vi "Check mtcdt check sd card write test.vi"(6 "VISA resource name":refnum<visa-resource-name>="COM5", 7 "Passed so far":bool, 8 "error in (no error)":errorcluster) -> (0 "error out":errorcluster, 1 "Card response":string, 2 "Source Response":string, 4 "VISA Refnum out":refnum<visa-resource-name>, 5 "Passed?":bool)   [LabVIEW 2024]
panel:
  out "Found sd card?":bool
  out "dest cksum":string
  out "src cksum":string
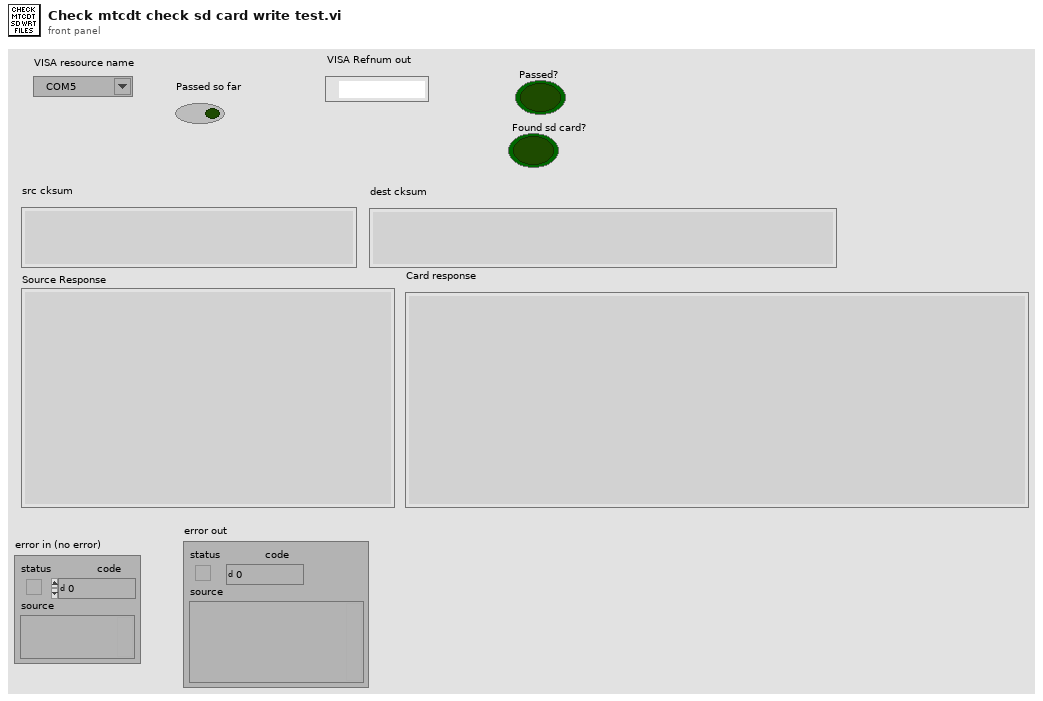
[diagram p1: front panel]
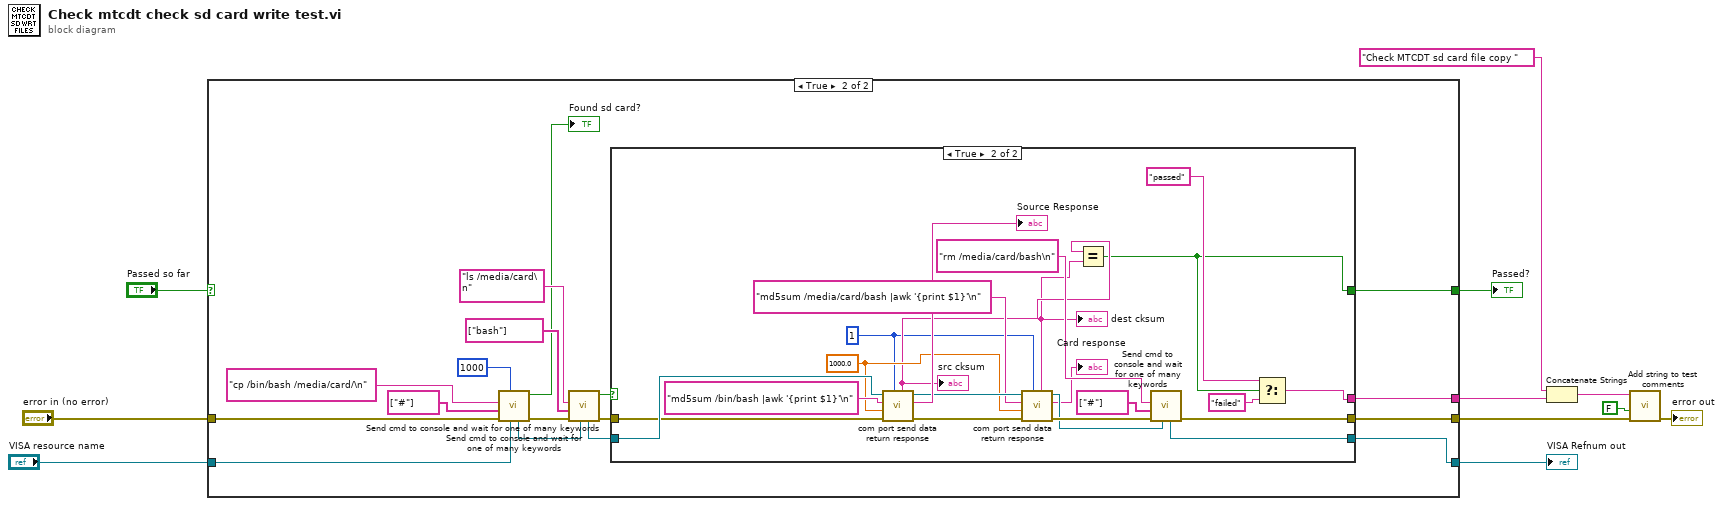
[diagram p0: block diagram]
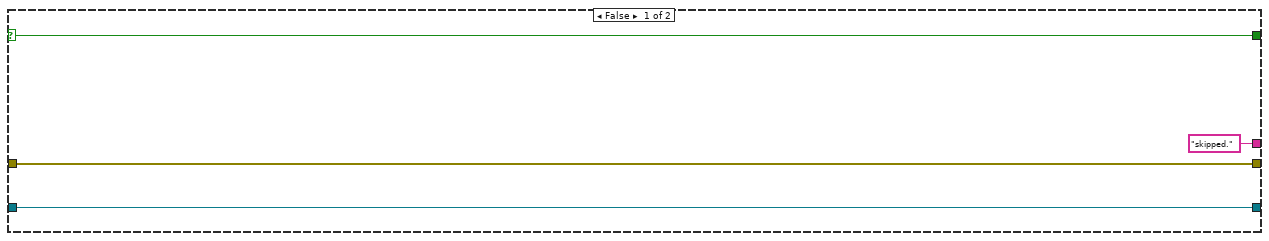
[diagram p2: hidden frame]
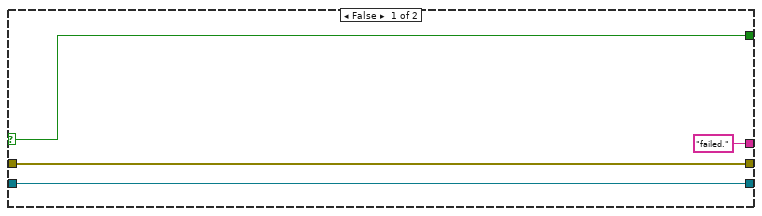
[diagram p3: hidden frame]
diagram:
  n1 = case shown="True" "Passed so far" {
    selector: "Passed so far" -> [w15 _]
    tunnel: "error in (no error)" -> [w14 w32]
    tunnel: [w14 w20] -> w2
    tunnel: "VISA resource name" -> [w13 w30]
    tunnel: [w15 w19] -> w6
    tunnel: [w13 w21] -> w3
    tunnel: ["skipped." w16] -> w1
    frame False {
    }
    frame True {
      n2 = call "Send cmd to console and wait for one of many keywords.vi"("VISA resource name"=w30, "Timeout (1000 mSecs)"=u32 1000 ("Timeout (mSecs)"), "error in (no error)"=w32, "Wait for keywords"=string[] ["#"], "write buffer"="cp /bin/bash /media/card/\n") -> ("error out"=w18:errorcluster, "Found key?"=→"Found sd card?":bool, "VISA Refnum out"=w27:refnum<visa-resource-name>)  [unwired: 2 in, 2 out]
      n3 = call "Send cmd to console and wait for one of many keywords.vi"("VISA resource name"=w27, "error in (no error)"=w18, "Wait for keywords"=string[] ["bash"], "write buffer"="ls /media/card\n") -> ("error out"=w23:errorcluster, "Found key?"=w24:bool, "VISA Refnum out"=w22:refnum<visa-resource-name>)  [unwired: 3 in, 2 out]
      n4 = case shown="True" w24 {
        selector: w24 -> [w34 _]
        tunnel: w23 -> [w36 w54]
        tunnel: w22 -> [w35 w55]
        tunnel: [w36 w57] -> w20
        tunnel: [w34 w38] -> w19
        tunnel: [w35 w56] -> w21
        tunnel: ["failed." w37] -> w16
        frame False {
        }
        frame True {
          w46 = u32 1 ("Return line number")
          w48 = 1000.0 ("Wait Msecs for response")
          n5 = call "com port send data return response.vi"("Return line number"=w46, "error in (no error)"=w54, "Wait Msecs for response"=w48, "Send data"="md5sum /bin/bash |awk '{print $1}'\n", "VISA resource name"=w55) -> ("error out"=w51:errorcluster, "response"=→"Source Response":string, "VISA resource name out"=w50:refnum<visa-resource-name>, "Response Line"=w47:string)  [unwired: 2 in, 1 out]
          "src cksum" <- w47
          n6 = call "com port send data return response.vi"("Return line number"=w46, "error in (no error)"=w51, "Wait Msecs for response"=w48, "Send data"="md5sum /media/card/bash |awk '{print $1}'\n", "VISA resource name"=w50) -> ("error out"=w44:errorcluster, "response"=→"Card response":string, "VISA resource name out"=w43:refnum<visa-resource-name>, "Response Line"=w45:string)  [unwired: 2 in, 1 out]
          "dest cksum" <- w45
          n7 = Equal?(x=w47, y=w45) -> (x = y?=w38:bool)
          n8 = call "Send cmd to console and wait for one of many keywords.vi"("VISA resource name"=w43, "error in (no error)"=w44, "Wait for keywords"=string[] ["#"], "write buffer"="rm /media/card/bash\n") -> ("error out"=w57:errorcluster, "VISA Refnum out"=w56:refnum<visa-resource-name>)  [unwired: 3 in, 3 out]
          n9 = Select(t="passed", s=w38, f="failed") -> (s? t:f=w37:string)
        }
      }
    }
  }
  "Passed?" <- w6
  "VISA Refnum out" <- w3
  n10 = Concatenate Strings("Check MTCDT sd card file copy " ("string"), w1) -> (w9:string)
  n11 = call "Add string to test comments.vi"("error in (no error)"=w2, "New Section (y)?"=FALSE, "Comments"=w9) -> ("error out"=→"error out":errorcluster)  [unwired: 7 in, 1 out]
